vi "Intro-CheckConnection.vi"() -> ()   [LabVIEW 2017]
doc: "This example demonstrates how to establish a connection to SPC modules.\n\ninfo@becker-hickl.com"
uses:
  SPC_Wrappers/SPC_Controls/SPCModInfo.ctl
  SPC_Wrappers/SPC_Controls/ModuleType.ctl
  SPC_Wrappers/SPC_Controls/ModuleTypes.ctl
panel:
  in  "Modul Type to Simulate":T1 items=["Hardware Modus"=0, "SPC-600 Simulation"=600, "SPC-630 Simulation"=630, "SPC-700  Simulation"=700, "SPC-730  Simulation"=730, "SPC-130  Simulation"=130, "SPC-830  Simulation"=830, "SPC-140  Simulation"=140, "SPC-930  Simulation"=930, "DPC-230  Simulation"=230, "SPC-150  Simulation"=150, "SPC-150 N  Simulation"=151, "SPC-150 NX  Simulation"=152, "SPC-130 EM  Simulation"=131, "SPC-130 EMN  Simulation"=132, "SPC-130 IN Simulation"=135, "SPC-130 INX Simulation"=136, "SPC-130 INXX Simulation"=137, "SPC-160  Simulation"=160, "SPC-160 X  Simulation"=161, "SPC-160 PCIE  Simulation"=162, "SPC-180 Simulation"=180, "SPC-181 Simulation"=181, "SPC-182 Simulation"=182, "SPC-185 Simulation"=185, "SPC-186 Simulation"=186, "SPC-187 Simulation"=187, "DPC-330  Simulation"=330, "DPC-590  Simulation"=590, "TDC-104 Simulation"=104, "TDC-004 Simulation"=4, "TDC-106 Simulation"=106]
  out "Serial Number":string[](array[string])
  out "Active Module No":i16[](array[numeric])
  out "Used Model Array":T2[](array[typedef]) {"Bus Number" min=-1 max=255 step=1; "Base I/O Addr" format="%.0x"; "Init Status" min=-10 max=0 step=1; "in Use" min=-1 max=1 step=1; "Slot Number" min=-1 max=255 step=1; "Module Type" items=["SPC-600"=600, "SPC-630"=630, "SPC-700"=700, "SPC-730"=730, "SPC-130"=130, "SPC-830"=830, "SPC-140"=140, "SPC-930"=930, "DPC-230"=230, "SPC-150"=150, "SPC-150 N"=151, "SPC-150 NX"=152, "SPC-130 EM"=131, "SPC-130 EMN"=132, "SPC-130IN"=135, "SPC-130INX"=136, "SPC-130INXX"=137, "SPC-160"=160, "SPC-160 X"=161, "SPC-160 PCIE"=162, "SPC-180 N"=180, "SPC-180 NX"=181, "SPC-180 NXX"=182, "SPC-180 N-USB"=185, "SPC-180 NX-USB"=186, "SPC-180 NXX-USB"=187, "SPC-QC-104"=104, "SPC-QC-004"=4, "SPC-QC-106"=106, "DPC-330"=330, "PMS-800"=800, "SPC-590"=590, "Simulation"=-1]}
  # "This example demonstrates how to establish a connection to SPC modules."
  # "(c) 2022 Becker & Hickl GmbH\n     All Rights Reserved."
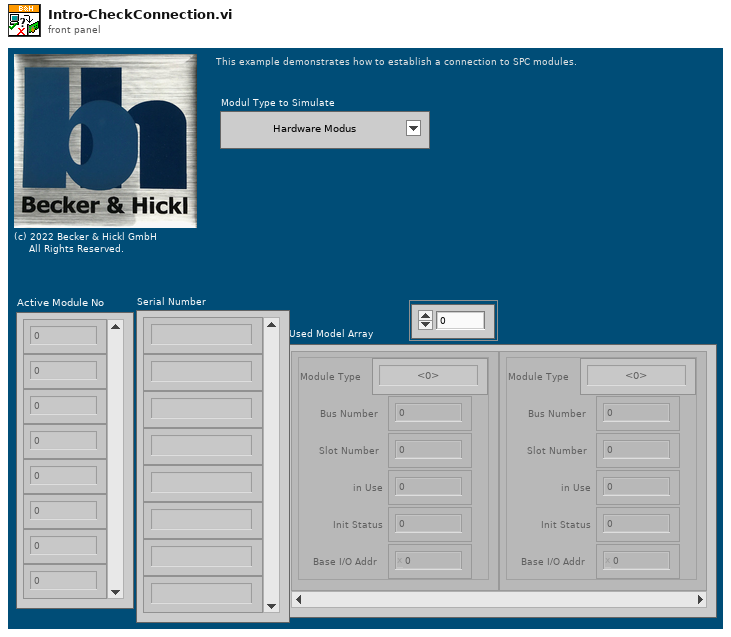
[diagram p1: front panel]
types:
  T1 = typedef "ModuleTypes.ctl" = i16
  T2 = typedef "SPCModInfo.ctl" = cluster{"Module Type":T3, "Bus Number":i16, "Slot Number":i16, "in Use":i16, "Init Status":i16, "Base I/O Addr":u16}
  T3 = typedef "ModuleType.ctl" = i16
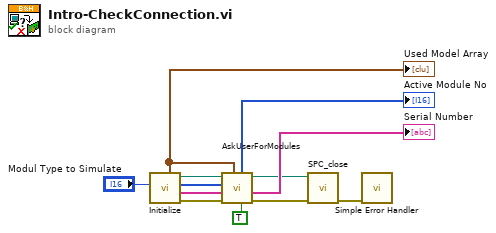
[diagram p0: block diagram]
diagram:
  n1 = call "Initialize.vi"("Modul Type to Simulate"="Modul Type to Simulate") -> ("ErrorOut"=w6:errorcluster, "SerialNumbersArray"=w10:string[], "ModuleNoArray"=w11:i16[], "DLL Path"=w7:path, "SPCModulesArray"=w4:T2[])  [unwired: 6 in]
  "Used Model Array" <- w4
  n2 = call "AskUserForModules.vi"("MultiModule"=TRUE, "SPCModulesArray"=w4, "Error In"=w6, "Serial Number"=w10, "ModuleNoArray"=w11, "DLL Path"=w7) -> ("Error Out"=w1:errorcluster, "ActiveSerialNumbers"=→"Serial Number":string[], "DLL Path"=w2:path, "ActiveModuleNo"=→"Active Module No":i16[])  [unwired: 1 in, 1 out]
  n3 = call "SPC_close.vi"("Error In"=w1, "DLL Path"=w2) -> ("Error Out"=w12:errorcluster)  [unwired: 8 in, 1 out]
  n4 = call <vilib>:"Simple Error Handler.vi"("error in (no error)"=w12) -> ()  [unwired: 4 in, 5 out]
